vi "Make Details Tags.vi"(2 "Details":T2={"ImageDescription"="", "XResolution"=0.0, "YResolution"=0.0, "ResolutionUnit"=enum."Inch", "PhotometricInterpretation"=0, "Compression"=enum."None", "PageName"="", "DocumentName"=""} {"PhotometricInterpretation" items=["PHOTOMETRIC_MINISWHITE"=0, "PHOTOMETRIC_MINISBLACK"=1, "PHOTOMETRIC_RGB"=2, "PHOTOMETRIC_PALETTE"=3, "PHOTOMETRIC_MASK"=4, "PHOTOMETRIC_SEPARATED"=5, "PHOTOMETRIC_YCBCR"=6, "PHOTOMETRIC_CIELAB"=8, "PHOTOMETRIC_ICCLAB"=9, "PHOTOMETRIC_ITULAB"=10, "PHOTOMETRIC_LOGL"=32844, "PHOTOMETRIC_LOGLUV"=32845, "CFA"=32803, "LinearRaw"=34892, "DEPTH"=51177]}, 3 "IFD Baseline":T1 {"SampleFormat" items=["UINT"=1, "INT"=2, "FP"=3, "VOID"=4, "COMPLEXINT"=5, "COMPLEXFP"=6]; "NewSubFileType" items=["FILETYPE_REDUCEDIMAGE"=1, "FILETYPE_PAGE"=2, "FILETYPE_MASK"=4]; "Compression" items=["COMPRESSION_NONE"=1, "COMPRESSION_CCITTRLE"=2, "COMPRESSION_CCITTFAX3"=3, "COMPRESSION_CCITTFAX4"=4, "COMPRESSION_LZW"=5, "COMPRESSION_OJPEG"=6, "COMPRESSION_JPEG"=7, "COMPRESSION_NEXT"=32766, "COMPRESSION_CCITTRLEW"=32771, "COMPRESSION_PACKBITS"=32773, "COMPRESSION_THUNDERSCAN"=32809, "COMPRESSION_IT8CTPAD"=32895, "COMPRESSION_IT8LW"=32896, "COMPRESSION_IT8MP"=32897, "COMPRESSION_IT8BL"=32898, "COMPRESSION_PIXARFILM"=32908, "COMPRESSION_PIXARLOG"=32909, "COMPRESSION_DEFLATE"=32946, "COMPRESSION_ADOBE_DEFLATE"=8, "COMPRESSION_DSC"=32947, "COMPRESSION_JBIG"=34661, "COMPRESSION_SGILOG"=34676, "COMPRESSION_SGILOG24"=34677, "COMPRESSION_JP2000"=34712]; "PhotometricInterpretation" items=["PHOTOMETRIC_MINISWHITE"=0, "PHOTOMETRIC_MINISBLACK"=1, "PHOTOMETRIC_RGB"=2, "PHOTOMETRIC_PALETTE"=3, "PHOTOMETRIC_MASK"=4, "PHOTOMETRIC_SEPARATED"=5, "PHOTOMETRIC_YCBCR"=6, "PHOTOMETRIC_CIELAB"=8, "PHOTOMETRIC_ICCLAB"=9, "PHOTOMETRIC_ITULAB"=10, "PHOTOMETRIC_LOGL"=32844, "PHOTOMETRIC_LOGLUV"=32845, "CFA"=32803, "LinearRaw"=34892, "DEPTH"=51177]; "ResolutionUnit" items=["RESUNIT_NONE"=1, "RESUNIT_INCH"=2, "RESUNIT_CENTIMETER"=3]}) -> (0 "Tags":cluster{"name":string, "Variant":variant}[](array[cluster]), 1 "Modified IFD Baseline":T1 {"SampleFormat" items=["UINT"=1, "INT"=2, "FP"=3, "VOID"=4, "COMPLEXINT"=5, "COMPLEXFP"=6]; "NewSubFileType" items=["FILETYPE_REDUCEDIMAGE"=1, "FILETYPE_PAGE"=2, "FILETYPE_MASK"=4]; "Compression" items=["COMPRESSION_NONE"=1, "COMPRESSION_CCITTRLE"=2, "COMPRESSION_CCITTFAX3"=3, "COMPRESSION_CCITTFAX4"=4, "COMPRESSION_LZW"=5, "COMPRESSION_OJPEG"=6, "COMPRESSION_JPEG"=7, "COMPRESSION_NEXT"=32766, "COMPRESSION_CCITTRLEW"=32771, "COMPRESSION_PACKBITS"=32773, "COMPRESSION_THUNDERSCAN"=32809, "COMPRESSION_IT8CTPAD"=32895, "COMPRESSION_IT8LW"=32896, "COMPRESSION_IT8MP"=32897, "COMPRESSION_IT8BL"=32898, "COMPRESSION_PIXARFILM"=32908, "COMPRESSION_PIXARLOG"=32909, "COMPRESSION_DEFLATE"=32946, "COMPRESSION_ADOBE_DEFLATE"=8, "COMPRESSION_DSC"=32947, "COMPRESSION_JBIG"=34661, "COMPRESSION_SGILOG"=34676, "COMPRESSION_SGILOG24"=34677, "COMPRESSION_JP2000"=34712]; "PhotometricInterpretation" items=["PHOTOMETRIC_MINISWHITE"=0, "PHOTOMETRIC_MINISBLACK"=1, "PHOTOMETRIC_RGB"=2, "PHOTOMETRIC_PALETTE"=3, "PHOTOMETRIC_MASK"=4, "PHOTOMETRIC_SEPARATED"=5, "PHOTOMETRIC_YCBCR"=6, "PHOTOMETRIC_CIELAB"=8, "PHOTOMETRIC_ICCLAB"=9, "PHOTOMETRIC_ITULAB"=10, "PHOTOMETRIC_LOGL"=32844, "PHOTOMETRIC_LOGLUV"=32845, "CFA"=32803, "LinearRaw"=34892, "DEPTH"=51177]; "ResolutionUnit" items=["RESUNIT_NONE"=1, "RESUNIT_INCH"=2, "RESUNIT_CENTIMETER"=3]})   [LabVIEW 2020, in "LV Tiff.lvlib"]
uses:
  LV Tiff.lvlib
  Tiff Page Details.ctl
  Baseline Tags 1.ctl
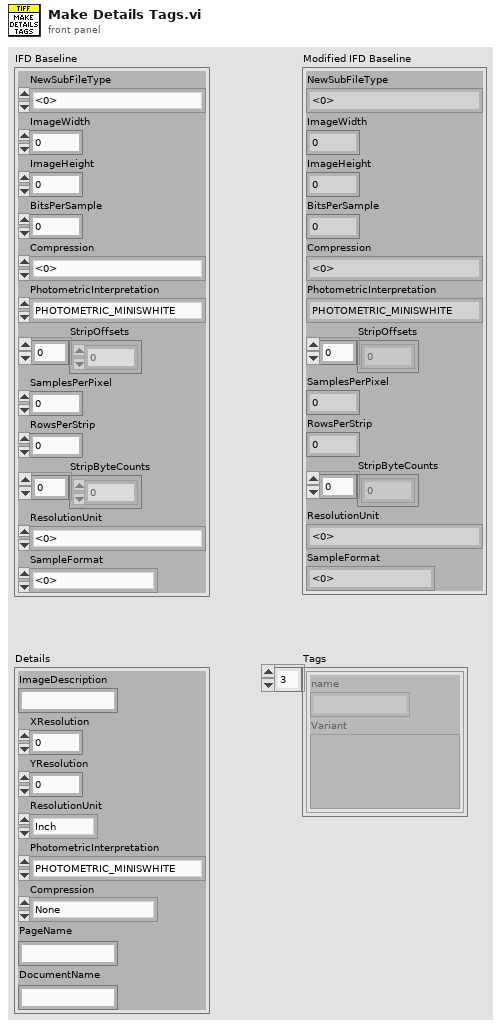
[diagram p1: front panel]
types:
  T1 = typedef "LV Tiff.lvlib/Baseline Tags 1.ctl" = cluster{"NewSubFileType":u32, "ImageWidth":u32, "ImageHeight":u32, "BitsPerSample":u16, "Compression":u16, "PhotometricInterpretation":u16, "StripOffsets":u32[], "SamplesPerPixel":u16, "RowsPerStrip":u32, "StripByteCounts":u32[], "ResolutionUnit":u16, "SampleFormat":u16}
  T2 = typedef "LV Tiff.lvlib/Tiff Page Details.ctl" = cluster{"ImageDescription":string, "XResolution":dbl, "YResolution":dbl, "ResolutionUnit":enum16{"None", "Inch", "Centimeter"}, "PhotometricInterpretation":u16, "Compression":enum16{"None", "Deflate", "JPEG"}, "PageName":string, "DocumentName":string}
  T3 = cluster{string, "ResolutionUnit":enum16{"None", "Inch", "Centimeter"}}
  T4 = cluster{string, "ResolutionUnit":enum16{"None", "Inch", "Centimeter"}}[]
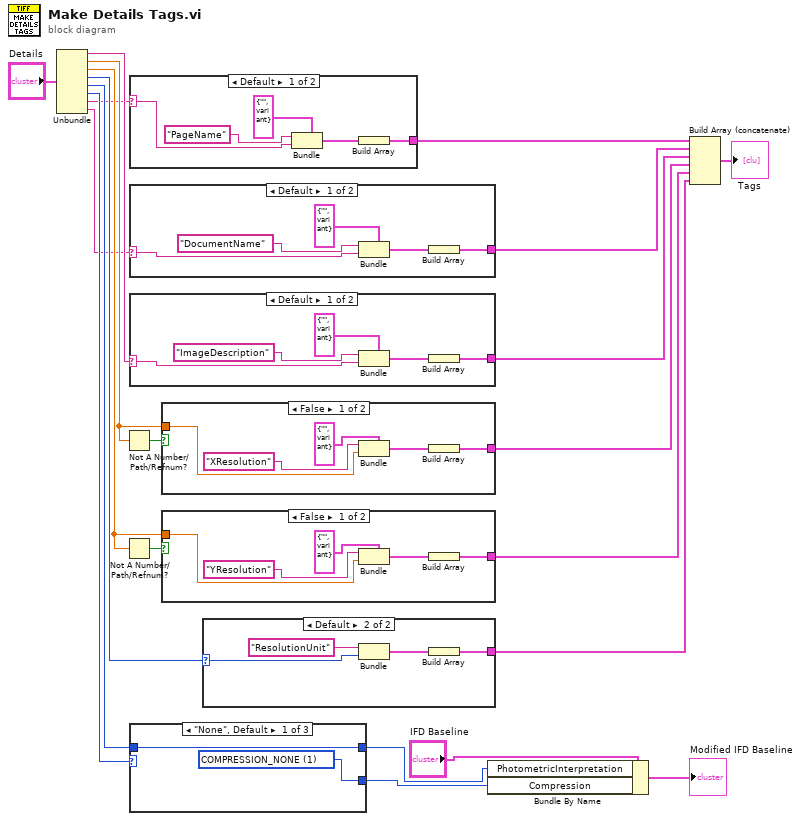
[diagram p0: block diagram]
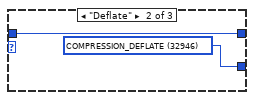
[diagram p5: hidden frame]
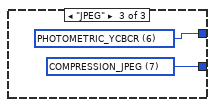
[diagram p6: hidden frame]
diagram:
  n1 = Unbundle("Details") -> ("ImageDescription"=w17:string, "XResolution"=w19:dbl, "YResolution"=w21:dbl, "ResolutionUnit"=w8:enum16{"None", "Inch", "Centimeter"}, "PhotometricInterpretation"=w13:u16, "Compression"=w12:enum16{"None", "Deflate", "JPEG"}, "PageName"=w4:string, "DocumentName"=w3:string)
  n2 = Not A Number/Path/Refnum?(number/path/refnum=w19) -> (NaN/Path/Refnum?=w18:bool)
  n3 = Not A Number/Path/Refnum?(number/path/refnum=w21) -> (NaN/Path/Refnum?=w20:bool)
  n4 = case shown="Default" w4 {
    selector: w4 -> [w24 _]
    tunnel: [w23 _] -> w1
    frame Default {
      n5 = Bundle(cluster=cluster{"name":string, "Variant":variant} {"name"="", "Variant"=variant}, "name"="PageName", "Variant"=w24) -> (w26:cluster{"name":string, "Variant":variant})
      n6 = Build Array(w26) -> (w23:cluster{"name":string, "Variant":variant}[])
    }
    frame "\u0000" {
    }
  }
  n7 = case shown="Default" w3 {
    selector: w3 -> [w29 _]
    tunnel: [w28 _] -> w2
    frame Default {
      n8 = Bundle(cluster=cluster{"name":string, "Variant":variant} {"name"="", "Variant"=variant}, "name"="DocumentName", "Variant"=w29) -> (w31:cluster{"name":string, "Variant":variant})
      n9 = Build Array(w31) -> (w28:cluster{"name":string, "Variant":variant}[])
    }
    frame "\u0000" {
    }
  }
  n10 = case shown="Default" w17 {
    selector: w17 -> [w34 _]
    tunnel: [w33 _] -> w6
    frame Default {
      n11 = Bundle(cluster=cluster{"name":string, "Variant":variant} {"name"="", "Variant"=variant}, "name"="ImageDescription", "Variant"=w34) -> (w36:cluster{"name":string, "Variant":variant})
      n12 = Build Array(w36) -> (w33:cluster{"name":string, "Variant":variant}[])
    }
    frame "\u0000" {
    }
  }
  n13 = case shown="\"None\", Default" w12 {
    tunnel: [w39 w41 w43] -> w15
    tunnel: [w38 w40 w42] -> w14
    tunnel: w13 -> [w38 w40 _]
    frame "None", Default {
      w39 = u16 1 items=["COMPRESSION_NONE"=1, "COMPRESSION_CCITTRLE"=2, "COMPRESSION_CCITTFAX3"=3, "COMPRESSION_CCITTFAX4"=4, "COMPRESSION_LZW"=5, "COMPRESSION_OJPEG"=6, "COMPRESSION_JPEG"=7, "COMPRESSION_NEXT"=32766, "COMPRESSION_CCITTRLEW"=32771, "COMPRESSION_PACKBITS"=32773, "COMPRESSION_THUNDERSCAN"=32809, "COMPRESSION_IT8CTPAD"=32895, "COMPRESSION_IT8LW"=32896, "COMPRESSION_IT8MP"=32897, "COMPRESSION_IT8BL"=32898, "COMPRESSION_PIXARFILM"=32908, "COMPRESSION_PIXARLOG"=32909, "COMPRESSION_DEFLATE"=32946, "COMPRESSION_ADOBE_DEFLATE"=8, "COMPRESSION_DSC"=32947, "COMPRESSION_JBIG"=34661, "COMPRESSION_SGILOG"=34676, "COMPRESSION_SGILOG24"=34677, "COMPRESSION_JP2000"=34712] ("Compression")
    }
    frame "Deflate" {
      w41 = u16 32946 items=["COMPRESSION_NONE"=1, "COMPRESSION_CCITTRLE"=2, "COMPRESSION_CCITTFAX3"=3, "COMPRESSION_CCITTFAX4"=4, "COMPRESSION_LZW"=5, "COMPRESSION_OJPEG"=6, "COMPRESSION_JPEG"=7, "COMPRESSION_NEXT"=32766, "COMPRESSION_CCITTRLEW"=32771, "COMPRESSION_PACKBITS"=32773, "COMPRESSION_THUNDERSCAN"=32809, "COMPRESSION_IT8CTPAD"=32895, "COMPRESSION_IT8LW"=32896, "COMPRESSION_IT8MP"=32897, "COMPRESSION_IT8BL"=32898, "COMPRESSION_PIXARFILM"=32908, "COMPRESSION_PIXARLOG"=32909, "COMPRESSION_DEFLATE"=32946, "COMPRESSION_ADOBE_DEFLATE"=8, "COMPRESSION_DSC"=32947, "COMPRESSION_JBIG"=34661, "COMPRESSION_SGILOG"=34676, "COMPRESSION_SGILOG24"=34677, "COMPRESSION_JP2000"=34712] ("Compression")
    }
    frame "JPEG" {
      w42 = u16 6 items=["PHOTOMETRIC_MINISWHITE"=0, "PHOTOMETRIC_MINISBLACK"=1, "PHOTOMETRIC_RGB"=2, "PHOTOMETRIC_PALETTE"=3, "PHOTOMETRIC_MASK"=4, "PHOTOMETRIC_SEPARATED"=5, "PHOTOMETRIC_YCBCR"=6, "PHOTOMETRIC_CIELAB"=8, "PHOTOMETRIC_ICCLAB"=9, "PHOTOMETRIC_ITULAB"=10, "PHOTOMETRIC_LOGL"=32844, "PHOTOMETRIC_LOGLUV"=32845, "CFA"=32803, "LinearRaw"=34892, "DEPTH"=51177] ("PhotometricInterpretation")
      w43 = u16 7 items=["COMPRESSION_NONE"=1, "COMPRESSION_CCITTRLE"=2, "COMPRESSION_CCITTFAX3"=3, "COMPRESSION_CCITTFAX4"=4, "COMPRESSION_LZW"=5, "COMPRESSION_OJPEG"=6, "COMPRESSION_JPEG"=7, "COMPRESSION_NEXT"=32766, "COMPRESSION_CCITTRLEW"=32771, "COMPRESSION_PACKBITS"=32773, "COMPRESSION_THUNDERSCAN"=32809, "COMPRESSION_IT8CTPAD"=32895, "COMPRESSION_IT8LW"=32896, "COMPRESSION_IT8MP"=32897, "COMPRESSION_IT8BL"=32898, "COMPRESSION_PIXARFILM"=32908, "COMPRESSION_PIXARLOG"=32909, "COMPRESSION_DEFLATE"=32946, "COMPRESSION_ADOBE_DEFLATE"=8, "COMPRESSION_DSC"=32947, "COMPRESSION_JBIG"=34661, "COMPRESSION_SGILOG"=34676, "COMPRESSION_SGILOG24"=34677, "COMPRESSION_JP2000"=34712] ("Compression")
    }
  }
  n14 = case shown="False" w18 {
    tunnel: w19 -> [w45 _]
    tunnel: [w44 _] -> w5
    frame False {
      n15 = Bundle(cluster=cluster{"name":string, "Variant":variant} {"name"="", "Variant"=variant}, "name"="XResolution", "Variant"=w45) -> (w47:cluster{"name":string, "Variant":variant})
      n16 = Build Array(w47) -> (w44:cluster{"name":string, "Variant":variant}[])
    }
    frame True {
    }
  }
  n17 = case shown="False" w20 {
    tunnel: w21 -> [w50 _]
    tunnel: [w49 _] -> w22
    frame False {
      n18 = Bundle(cluster=cluster{"name":string, "Variant":variant} {"name"="", "Variant"=variant}, "name"="YResolution", "Variant"=w50) -> (w52:cluster{"name":string, "Variant":variant})
      n19 = Build Array(w52) -> (w49:cluster{"name":string, "Variant":variant}[])
    }
    frame True {
    }
  }
  n20 = case shown="Default" w8 {
    selector: w8 -> [_ w56]
    tunnel: [_ w54] -> w7
    frame "None" {
    }
    frame Default {
      n21 = Bundle("ResolutionUnit", "ResolutionUnit"=w56) -> (w55:T3)  [unwired: 1 in]
      n22 = Build Array(w55) -> (w54:T4)
    }
  }
  n23 = Bundle By Name(cluster="IFD Baseline", "PhotometricInterpretation"=w14, "Compression"=w15) -> (→"Modified IFD Baseline":T1)
  n24 = Build Array (concatenate)(w1, w2, w6, w5, w22, w7) -> (→"Tags":cluster{"name":string, "Variant":variant}[])
